vi "Vacuum Switch Panel1.vi"() -> ()   [LabVIEW 2020]
uses:
  Classes/Controller/Controller.lvclass
  Classes/Controller/I-O/I-O.lvclass
panel:
  out "Compression Sensor":bool
  out "Sensor Channel":dbl
  out "Sensor":bool
  out "sensor pin number":i32
  out "tray sensor":bool
  out "secondary valve sensor":bool
  out "primary valve sensor":bool
  in  "Turn on secondary vacuum":bool
  in  "turn on primary vacuum":bool
  in  "secure tray":bool
  out "Valve Channel":dbl
  in  "Type":enum16{"O ring Vac", "Baseplate Vac"}(ring)
  in  "Position":i32
  in  "Region":i32
  in  "On/Off":bool
  in  "Stop":bool
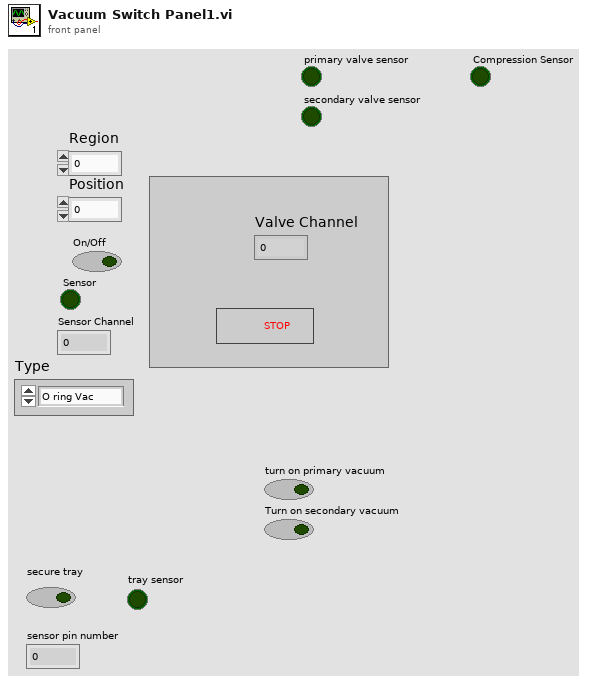
[diagram p1: front panel]
types:
  T1 = typedef "Controller.lvclass/Controllers.ctl" = cluster{"I-O.lvclass":refnum<class "I-O.lvclass">, "Gantry":refnum<k24>, "Dispenser":refnum<visa-resource-name>}
  T2 = typedef "I-O.lvclass/Pin Map.ctl" = cluster{"Region Valves":i32[], "Extra Valves":dbl[][][], "Tool Primary Valve":i32, "Tool Secondary Valve":i32, "Region Sensors":i32[], "Extra Sensors":dbl[][][], "Tool Primary Sensor":dbl, "Tool Secondary Sensor":dbl, "Compression Sensor":dbl, "5V":i32, "Dispenser Sensor":dbl}
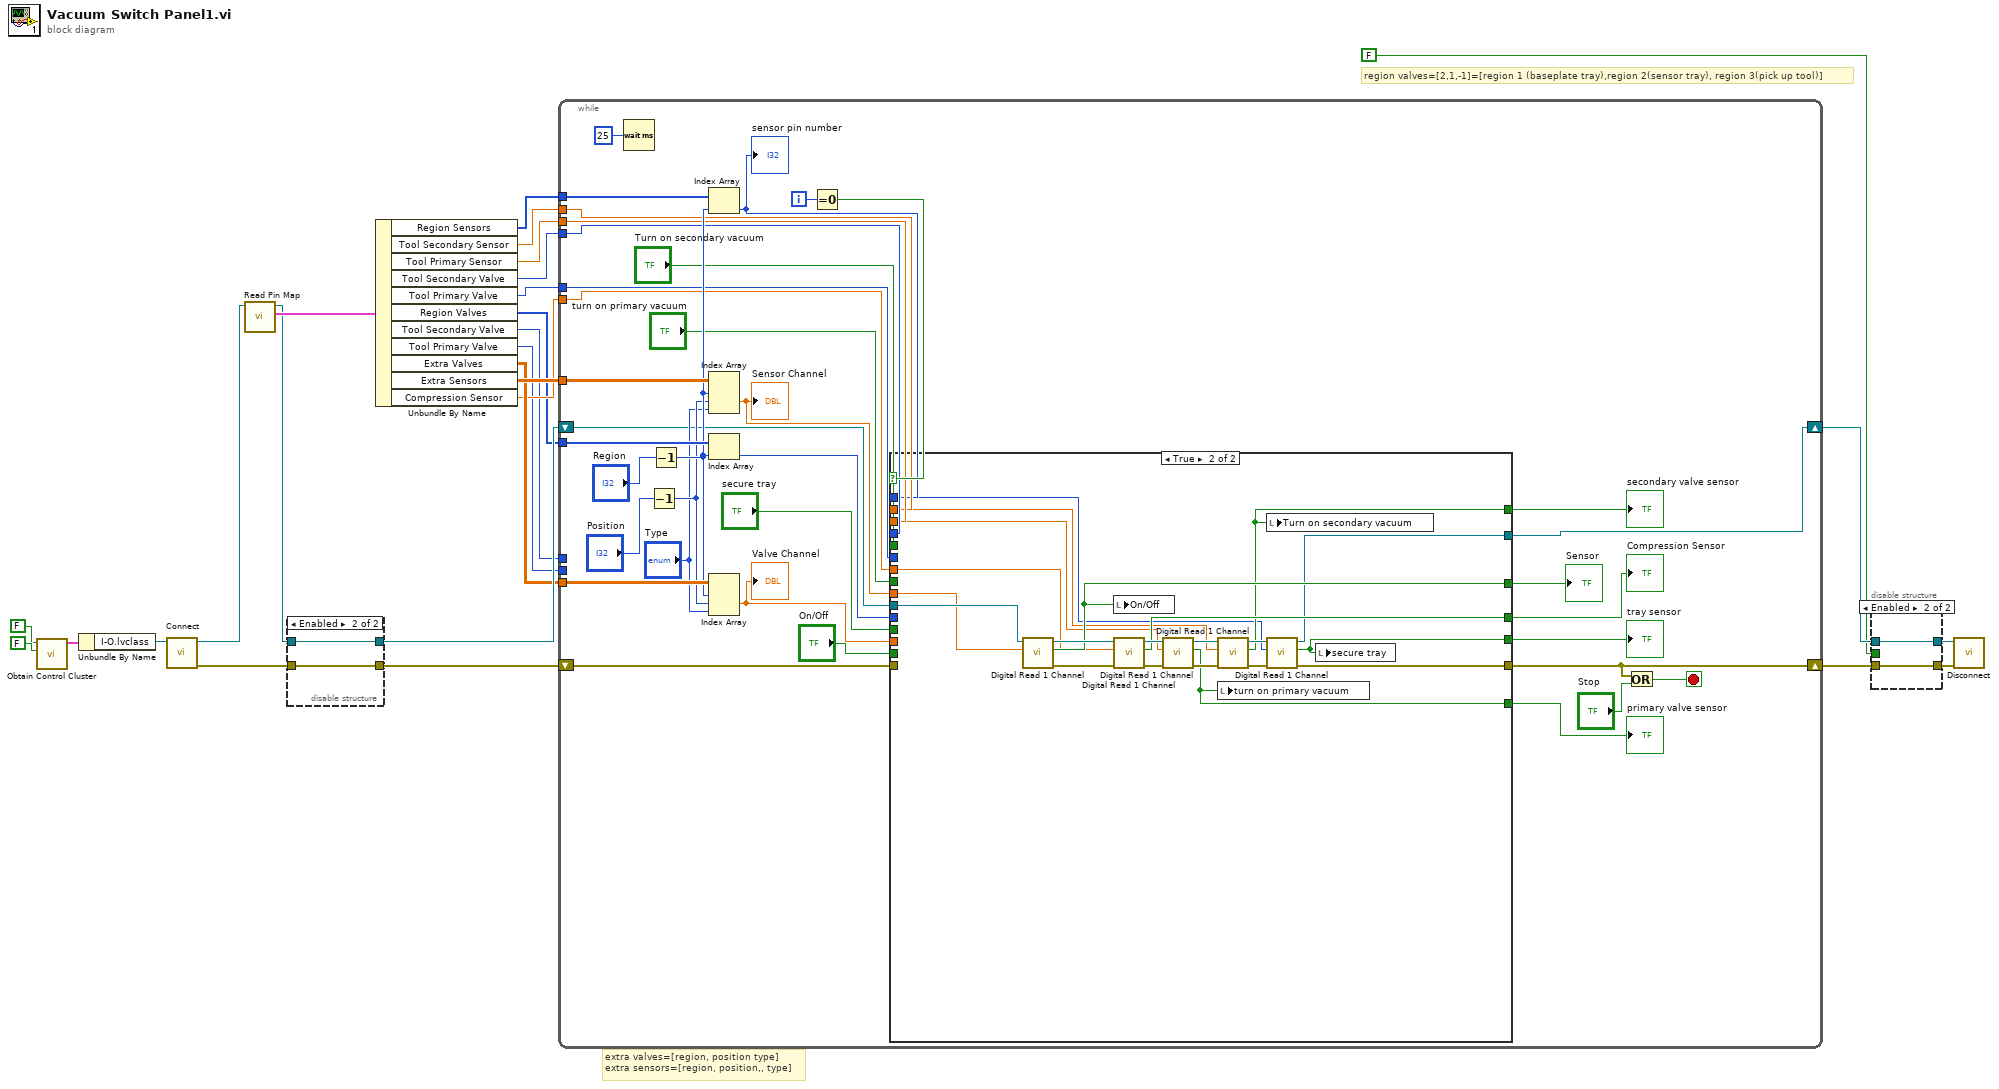
[diagram p0: block diagram]
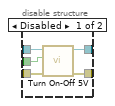
[diagram p2: hidden frame]
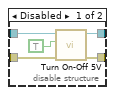
[diagram p3: hidden frame]
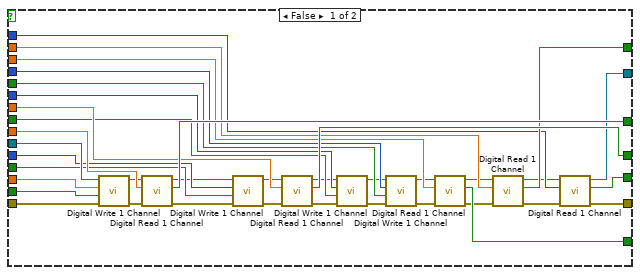
[diagram p4: hidden frame]
diagram:
  # "extra valves=[region, position type]\nextra sensors=[region, position,, type]"
  # "region valves=[2,1,-1]=[region 1 (baseplate tray),region 2(sensor tray), region 3(pick up tool)]"
  n1 = call "Obtain Control Cluster.vi"("Dispense"=FALSE, "Motion"=FALSE) -> ("Control Out"=w11:T1)  [unwired: 9 in]
  n2 = Unbundle By Name(w11) -> ("I-O.lvclass"=w10:refnum<class "I-O.lvclass">)
  n3 = call-dynamic "Connect.vi"("Controller in"=w10) -> ("error out"=w18:errorcluster, "Controller out"=w20:refnum<class "I-O.lvclass">)  [unwired: 9 in]
  n4 = call-dynamic "Read Pin Map.vi"("I-O in"=w20) -> ("Pin Map 2"=w22:T2, "I-O out"=w21:refnum<class "I-O.lvclass">)  [unwired: 8 in, 1 out]
  n5 = disable-structure shown="Enabled" {
    disable-tunnel: [w31 w33] -> w26
    disable-tunnel: w21 -> [w29 w33]
    disable-tunnel: w18 -> [w28 w32]
    disable-tunnel: [w27 w32] -> w17
    frame Disabled {
      n6 = call-dynamic "Turn On-Off 5V.vi"("error in (no error)"=w28, "Value"=TRUE, "I-O in"=w29) -> ("error out"=w27:errorcluster, "I-O out"=w31:refnum<class "I-O.lvclass">)  [unwired: 7 in]
    }
    frame Enabled {
    }
  }
  n7 = Unbundle By Name(w22) -> ("Region Sensors"=w1:i32[], "Tool Secondary Sensor"=w2:dbl, "Tool Primary Sensor"=w3:dbl, "Tool Secondary Valve"=w4:i32, "Tool Primary Valve"=w5:i32, "Region Valves"=w6:i32[], "Tool Secondary Valve"=w8:i32, "Tool Primary Valve"=w7:i32, "Extra Valves"=w14:dbl[][][], "Extra Sensors"=w19:dbl[][][], "Compression Sensor"=w9:dbl)
  n8 = while {
    shift-right: [w35] -> w24
    shift-left: w26 -> [w53]
    tunnel: w19 -> [w61]
    shift-right: [w37] -> w16
    shift-left: w17 -> [w55]
    tunnel: w14 -> [w62]
    tunnel: w9 -> [w48]
    tunnel: w8 -> [_]
    tunnel: w7 -> [_]
    tunnel: w6 -> [w64]
    tunnel: w5 -> [w45]
    tunnel: w4 -> [w43]
    tunnel: w3 -> [w42]
    tunnel: w2 -> [w40]
    tunnel: w1 -> [w63]
    i -> [w57]
    stop <- w67 stop-if-true
    n9 = Wait (ms)(milliseconds to wait=u32 25) -> ()  [unwired: 1 out]
    n10 = Decrement(x="Position") -> (x-1=w59:i32)
    n11 = Decrement(x="Region") -> (x-1=w60:i32)
    n12 = Index Array(array=w63, index=w60) -> (element=w38:i32)
    "sensor pin number" <- w38
    n13 = Index Array(array=w61, index (dim 0)=w60, index (dim 1)=w59, index (dim 2)="Type") -> (element=w52:dbl)
    "Sensor Channel" <- w52
    n14 = Index Array(array=w64, index=w60) -> (element=w49:i32)
    n15 = Index Array(array=w62, index (dim 0)=w60, index (dim 1)=w59, index (dim 2)="Type") -> (element=w54:dbl)
    "Valve Channel" <- w54
    n16 = Equal To 0?(x=w57) -> (x = 0?=w56:bool)
    n17 = case shown="True" w56 {
      tunnel: w55 -> [w107 _]
      tunnel: w54 -> [w106 _]
      tunnel: w53 -> [w105 w120]
      tunnel: w52 -> [w103 w118]
      tunnel: [w101 w119] -> w51
      tunnel: "secure tray" -> [w99 _]
      tunnel: w49 -> [w98 _]
      tunnel: w48 -> [w95 w116]
      tunnel: [w93 w117] -> w47
      tunnel: "turn on primary vacuum" -> [w91 _]
      tunnel: w45 -> [w90 _]
      tunnel: "Turn on secondary vacuum" -> [w87 _]
      tunnel: w43 -> [w86 _]
      tunnel: w42 -> [w83 w115]
      tunnel: [w81 w114] -> w41
      tunnel: w40 -> [w79 w113]
      tunnel: [w77 w112] -> w39
      tunnel: w38 -> [w75 w111]
      tunnel: [w73 w108] -> w37
      tunnel: [w72 w110] -> w36
      tunnel: [w71 w109] -> w35
      tunnel: "On/Off" -> [w70 _]
      frame False {
        n18 = call-dynamic "Digital Write 1 Channel.vi"("error constant"=w107, "Value"=w70, "Channel"=w106, "I-O.lvclass"=w105) -> ("error IO"=w104:errorcluster, "I-O.lvclass 2"=w102:refnum<class "I-O.lvclass">)  [unwired: 6 in]
        n19 = call-dynamic "Digital Read 1 Channel.vi"("error in (no error)"=w104, "Read"=w103, "I-O in"=w102) -> ("error out"=w100:errorcluster, "Value"=w101:bool, "I-O out"=w97:refnum<class "I-O.lvclass">)  [unwired: 6 in]
        n20 = call-dynamic "Digital Write 1 Channel.vi"("error constant"=w100, "Value"=w99, "Channel"=w98, "I-O.lvclass"=w97) -> ("error IO"=w96:errorcluster, "I-O.lvclass 2"=w94:refnum<class "I-O.lvclass">)  [unwired: 6 in]
        n21 = call-dynamic "Digital Read 1 Channel.vi"("error in (no error)"=w96, "Read"=w95, "I-O in"=w94) -> ("error out"=w92:errorcluster, "Value"=w93:bool, "I-O out"=w89:refnum<class "I-O.lvclass">)  [unwired: 6 in]
        n22 = call-dynamic "Digital Write 1 Channel.vi"("error constant"=w92, "Value"=w91, "Channel"=w90, "I-O.lvclass"=w89) -> ("error IO"=w88:errorcluster, "I-O.lvclass 2"=w85:refnum<class "I-O.lvclass">)  [unwired: 6 in]
        n23 = call-dynamic "Digital Write 1 Channel.vi"("error constant"=w88, "Value"=w87, "Channel"=w86, "I-O.lvclass"=w85) -> ("error IO"=w84:errorcluster, "I-O.lvclass 2"=w82:refnum<class "I-O.lvclass">)  [unwired: 6 in]
        n24 = call-dynamic "Digital Read 1 Channel.vi"("error in (no error)"=w84, "Read"=w83, "I-O in"=w82) -> ("error out"=w80:errorcluster, "Value"=w81:bool, "I-O out"=w78:refnum<class "I-O.lvclass">)  [unwired: 6 in]
        n25 = call-dynamic "Digital Read 1 Channel.vi"("error in (no error)"=w80, "Read"=w79, "I-O in"=w78) -> ("error out"=w76:errorcluster, "Value"=w77:bool, "I-O out"=w74:refnum<class "I-O.lvclass">)  [unwired: 6 in]
        n26 = call-dynamic "Digital Read 1 Channel.vi"("error in (no error)"=w76, "Read"=w75, "I-O in"=w74) -> ("error out"=w73:errorcluster, "Value"=w72:bool, "I-O out"=w71:refnum<class "I-O.lvclass">)  [unwired: 6 in]
      }
      frame True {
        n27 = call-dynamic "Digital Read 1 Channel.vi"("Read"=w118, "I-O in"=w120) -> ("error out"=w125:errorcluster, "Value"=w119:bool, "I-O out"=w128:refnum<class "I-O.lvclass">)  [unwired: 7 in]
        n28 = local write "On/Off"(w119) -> ()
        n29 = call-dynamic "Digital Read 1 Channel.vi"("error in (no error)"=w125, "Read"=w116, "I-O in"=w128) -> ("error out"=w124:errorcluster, "Value"=w117:bool, "I-O out"=w127:refnum<class "I-O.lvclass">)  [unwired: 6 in]
        n30 = call-dynamic "Digital Read 1 Channel.vi"("error in (no error)"=w124, "Read"=w115, "I-O in"=w127) -> ("error out"=w123:errorcluster, "Value"=w114:bool, "I-O out"=w126:refnum<class "I-O.lvclass">)  [unwired: 6 in]
        n31 = call-dynamic "Digital Read 1 Channel.vi"("error in (no error)"=w123, "Read"=w113, "I-O in"=w126) -> ("error out"=w121:errorcluster, "Value"=w112:bool, "I-O out"=w122:refnum<class "I-O.lvclass">)  [unwired: 6 in]
        n32 = local write "turn on primary vacuum"(w114) -> ()
        n33 = local write "Turn on secondary vacuum"(w112) -> ()
        n34 = call-dynamic "Digital Read 1 Channel.vi"("error in (no error)"=w121, "Read"=w111, "I-O in"=w122) -> ("error out"=w108:errorcluster, "Value"=w110:bool, "I-O out"=w109:refnum<class "I-O.lvclass">)  [unwired: 6 in]
        n35 = local write "secure tray"(w110) -> ()
      }
    }
    "primary valve sensor" <- w41
    "secondary valve sensor" <- w39
    "tray sensor" <- w36
    "Sensor" <- w51
    "Compression Sensor" <- w47
    n36 = Or(x=w37, y="Stop") -> (x .or. y?=w67:bool)
  }
  n37 = disable-structure shown="Enabled" {
    disable-tunnel: [w133 w135] -> w25
    disable-tunnel: w24 -> [w132 w135]
    disable-tunnel: FALSE ("Value") -> [w131 _]
    disable-tunnel: w16 -> [w130 w134]
    disable-tunnel: [w129 w134] -> w15
    frame Disabled {
      n38 = call-dynamic "Turn On-Off 5V.vi"("error in (no error)"=w130, "Value"=w131, "I-O in"=w132) -> ("error out"=w129:errorcluster, "I-O out"=w133:refnum<class "I-O.lvclass">)  [unwired: 7 in]
    }
    frame Enabled {
    }
  }
  n39 = call-dynamic "Disconnect.vi"("error in (no error)"=w15, "I-O in"=w25) -> ()  [unwired: 8 in, 1 out]
